vi "FM Ch Read Multi Frm.vi"(0 "devId":i32, 1 "pBuffer":string, 2 "BytesReturned":u32, 5 "Channel":u8, 7 "FrameCnt":u32, 9 "BufSize":u32, 12 "FrmReturned":u32) -> (3 "pBuffer out":string, 4 "BytesReturned out":u32, 6 "function return":i32, 8 "devId out":i32, 14 "FrmReturned out":u32)   [LabVIEW 2013, in "CHR34XXX.lvlib"]
doc: "DLL BOOL __stdcall CHR34XXX_FM_Ch_RxMode(IN int devId,IN BYTE Channel,IN BYTE RxMode); DLL BOOL __stdcall CHR34XXX_FM_Ch_RxFrmCount(IN int devId,IN BYTE Channel,OUT DWORD *FrmCnt); DLL BOOL __stdcall CHR34XXX_FM_Ch_ReadFrm(IN int devId,IN BYTE Channel,IN DWORD BufSize,OUT BYTE *pBuffer,OUT DWORD *pReturned); DLL BYTE __stdcall CHR34XXX_FM_Ch_ReadRefreshFrm(IN int devId,IN BYTE Channel,IN DWORD BufSize,OUT BYTE *pBuffer,OUT DWORD *pReturned); DLL BOOL __stdcall CHR34XXX_FM_Ch_ReadMultiFrm(IN int devId,IN BYTE Channel,IN DWORD FrameCnt, IN DWORD BufSize,\n OUT BYTE *pBuffer, OUT DWORD *FrmReturned, OUT DWORD *BytesReturned);"
uses:
  CHR34XXX.lvlib
  CHR34XXX.dll
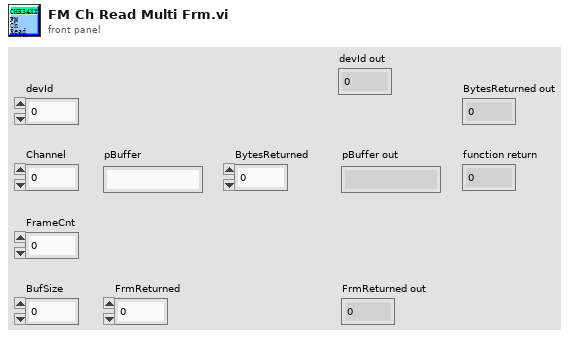
[diagram p1: front panel]
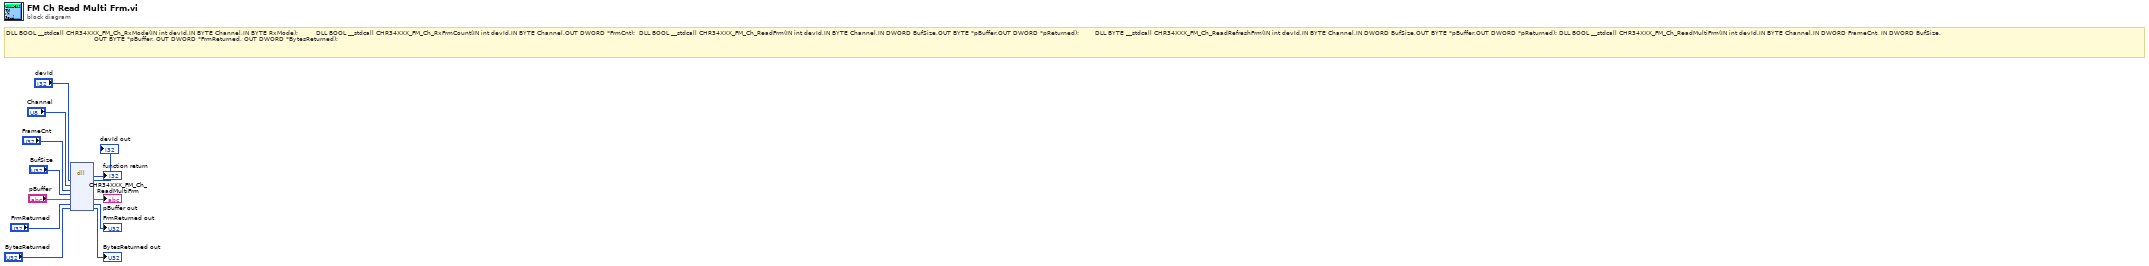
[diagram p0: block diagram]
diagram:
  # "DLL BOOL __stdcall CHR34XXX_FM_Ch_RxMode(IN int devId,IN BYTE Channel,IN BYTE RxMode);         DLL BOOL __stdcall CHR34XXX_FM_Ch_RxFrmCount(IN int devId,IN BYTE Channel,OUT DWORD *FrmCnt);  DLL BOOL __stdcall CHR34XXX_FM_Ch_ReadFrm(IN int devId,IN BYTE Channel,IN DWORD BufSize,OUT BYTE *pBuffer,OUT DWORD *pReturned);        DLL BYTE __stdcall CHR34XXX_FM_Ch_ReadRefreshFrm(IN int devId,IN BYTE Channel,IN DWORD BufSize,OUT BYTE *pBuffer,OUT DWORD *pReturned); DLL BOOL __stdcall CHR34XXX_FM_Ch_ReadMultiFrm(IN int devId,IN BYTE Channel,IN DWORD FrameCnt, IN DWORD BufSize,\n\t                                           OUT BYTE *pBuffer, OUT DWORD *FrmReturned, OUT DWORD *BytesReturned);"
  n1 = dll-call lib="C:/Users/Administrator/Desktop/CHR34XXX_lv/lv_lib/CHR34XXX.*" fn="CHR34XXX_FM_Ch_ReadMultiFrm"("devId"="devId", "Channel"="Channel", "FrameCnt"="FrameCnt", "BufSize"="BufSize", "pBuffer"="pBuffer", "FrmReturned"="FrmReturned", "BytesReturned"="BytesReturned") -> (→"function return":i32, "devId"=→"devId out":i32, "pBuffer"=→"pBuffer out":string, "FrmReturned"=→"FrmReturned out":u32, "BytesReturned"=→"BytesReturned out":u32)  [unwired: 6 in, 2 out]
